vi "Parse Data Out.vi"(0 "Raw Data In":string, 11 "Error In":errorcluster) -> (4 "Data Out":T1 {"CRC" format="%04x"; "Length" format="%02x"; "Command" format="%02x"; "Destination" format="%02x"; "Source" format="%02x"}, 8 "Raw Data Out":string, 15 "Error Out":errorcluster)   [LabVIEW 2023]
uses:
  library/GEA2_Toolkit.lvlib
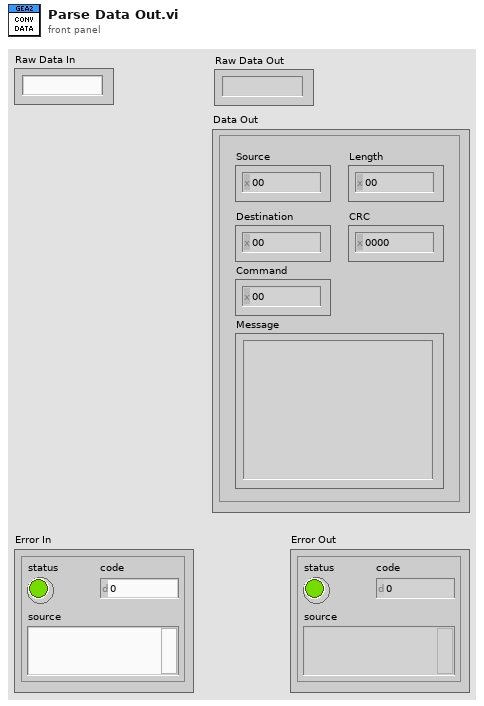
[diagram p1: front panel]
types:
  T1 = cluster{"Source":u8, "Destination":u8, "Command":u8, "Length":u8, "CRC":u16, "Message":string}
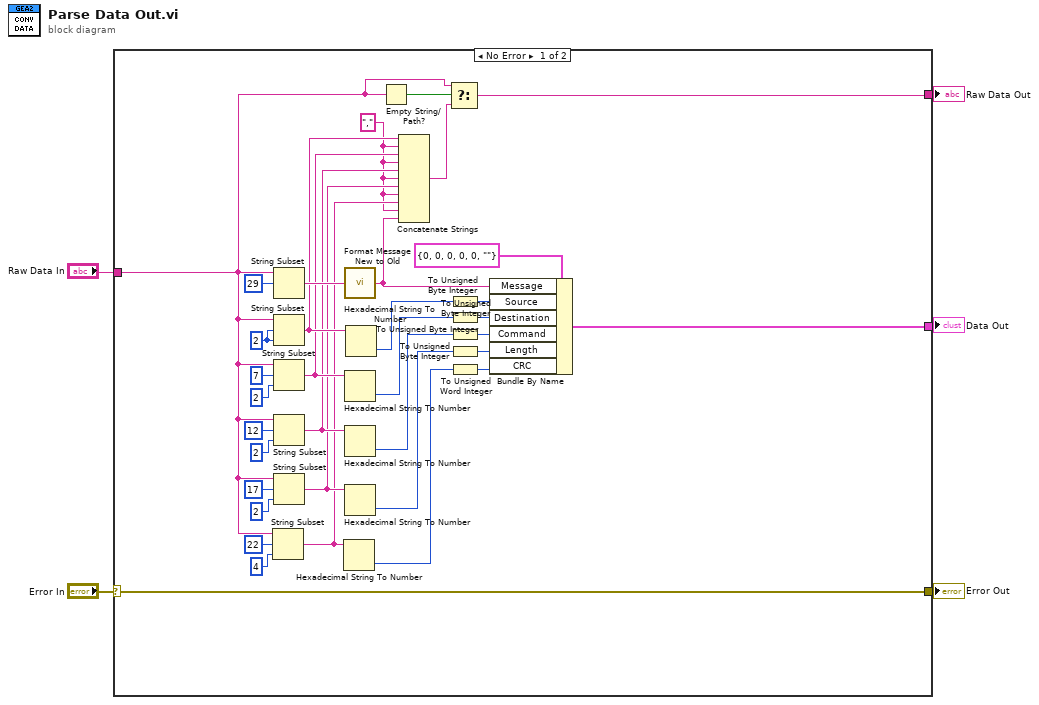
[diagram p0: block diagram]
diagram:
  n1 = case shown="No Error" "Error In" {
    selector: "Error In" -> [w35 w41]
    tunnel: [w35 w41] -> w4
    tunnel: [w32 _] -> w3
    tunnel: "Raw Data In" -> [w13 _]
    tunnel: [w11 _] -> w1
    frame No Error {
      w16 = "," ("string")
      w23 = 2 ("length (rest)")
      n2 = String Subset(string=w13, offset (0)=22, length (rest)=4 ("length (rest)")) -> (substring=w17:string)
      n3 = String Subset(string=w13, offset (0)=29) -> (substring=w22:string)  [unwired: 1 in]
      n4 = String Subset(string=w13, offset (0)=w23, length (rest)=w23) -> (substring=w21:string)
      n5 = String Subset(string=w13, offset (0)=7, length (rest)=2 ("length (rest)")) -> (substring=w20:string)
      n6 = String Subset(string=w13, offset (0)=12, length (rest)=2 ("length (rest)")) -> (substring=w19:string)
      n7 = String Subset(string=w13, offset (0)=17, length (rest)=2 ("length (rest)")) -> (substring=w18:string)
      n8 = Hexadecimal String To Number(string=w17) -> (number=w24:u32)  [unwired: 2 in, 1 out]
      n9 = call "Format Message New to Old.vi"("Raw Message In"=w22) -> ("Conv Message Out"=w15:string)  [unwired: 14 in]
      n10 = Hexadecimal String To Number(string=w20) -> (number=w10:u32)  [unwired: 2 in, 1 out]
      n11 = Hexadecimal String To Number(string=w19) -> (number=w34:u32)  [unwired: 2 in, 1 out]
      n12 = Hexadecimal String To Number(string=w18) -> (number=w28:u32)  [unwired: 2 in, 1 out]
      n13 = Hexadecimal String To Number(string=w21) -> (number=w9:u32)  [unwired: 2 in, 1 out]
      n14 = Empty String/Path?(string/path=w13) -> (empty?=w14:bool)
      n15 = Concatenate Strings(w21, w16, w20, w16, w19, w16, w18, w16, w17, w16, w15) -> (w12:string)
      n16 = Select(t=w13, s=w14, f=w12) -> (s? t:f=w11:string)
      n17 = To Unsigned Byte Integer(number=w9) -> (unsigned 8bit integer=w6:u8)
      n18 = To Unsigned Byte Integer(number=w10) -> (unsigned 8bit integer=w7:u8)
      n19 = To Unsigned Byte Integer(number=w34) -> (unsigned 8bit integer=w8:u8)
      n20 = To Unsigned Byte Integer(number=w28) -> (unsigned 8bit integer=w29:u8)
      n21 = To Unsigned Word Integer(number=w24) -> (unsigned 16bit integer=w27:u16)
      n22 = Bundle By Name(cluster=T1 {"Source"=0, "Destination"=0, "Command"=0, "Length"=0, "CRC"=0, "Message"=""} ("Data Out"), "Message"=w15, "Source"=w6, "Destination"=w7, "Command"=w8, "Length"=w29, "CRC"=w27) -> (w32:T1)
    }
    frame Error {
    }
  }
  "Error Out" <- w4
  "Data Out" <- w3
  "Raw Data Out" <- w1
